vi "File List Write Files.vi"(10 "Files":path[](array[path]), 11 "File List in":refnum<class "File List.lvclass">) -> (2 "Current file out":path, 3 "File List out":refnum<class "File List.lvclass">)   [LabVIEW 2011, in "COSYLib.lvlib" / "File List.lvclass"]
doc: "Sets the list of files.\nAny empty paths in the list are automatically removed.\nThe current file index is reset to the first file in the list.\nThe newly active file is returned."
uses:
  File List.lvclass
  File List.lvclass/File List.ctl
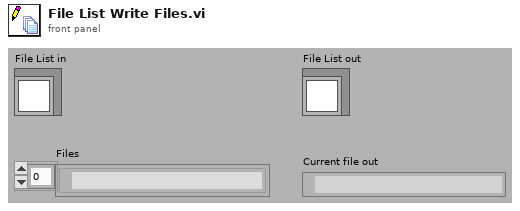
[diagram p1: front panel]
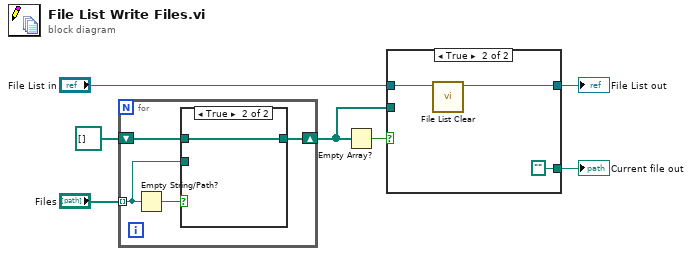
[diagram p0: block diagram]
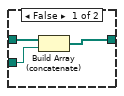
[diagram p2: hidden frame]
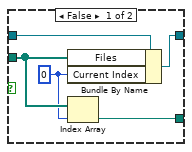
[diagram p3: hidden frame]
diagram:
  n1 = for {
    tunnel: "Files" -> [w10] mode=indexing
    shift-right: [w9] -> w2
    shift-left: path[] [] ("Files") -> [w8]
    n2 = Empty String/Path?(string/path=w10) -> (empty?=w11:bool)
    n3 = case shown="True" w11 {
      tunnel: w10 -> [w12 _]
      tunnel: [w13 w15] -> w9
      tunnel: w8 -> [w14 w15]
      frame False {
        n4 = Build Array (concatenate)(w14, w12) -> (w13:path[])
      }
      frame True {
      }
    }
  }
  n5 = Empty Array?(array=w2) -> (empty?=w7:bool)
  n6 = case shown="True" w7 {
    tunnel: "File List in" -> [w20 w23]
    tunnel: [w19 w22] -> w5
    tunnel: w2 -> [w18 _]
    tunnel: [w16 path ""] -> w1
    frame False {
      w17 = 0 ("Current Index")
      n7 = Bundle By Name(cluster=w20, "Files"=w18, "Current Index"=w17) -> (w19:refnum<class "File List.lvclass">)
      n8 = Index Array(array=w18, index=w17) -> (element=w16:path)
    }
    frame True {
      n9 = call "File List Clear.vi"("File List in"=w23) -> ("File List out"=w22:refnum<class "File List.lvclass">)  [unwired: 10 in]
    }
  }
  "File List out" <- w5
  "Current file out" <- w1
